vi "FRCts20_Backend_Competition_PPD_return.vi"(7 "Competition":T1, 8 "error in (no error)":errorcluster, 10 "rows affected":i32) -> (0 "error out":errorcluster, 3 "data string":string)   [LabVIEW 2014]
uses:
  FRCts20_Backend_API/FRCts20_Backend_API_Competition.ctl
  FRCts20_Backend_Engine.lvlib
  FRCts20_Backend_API/FRCts20_Backend_API.lvlib
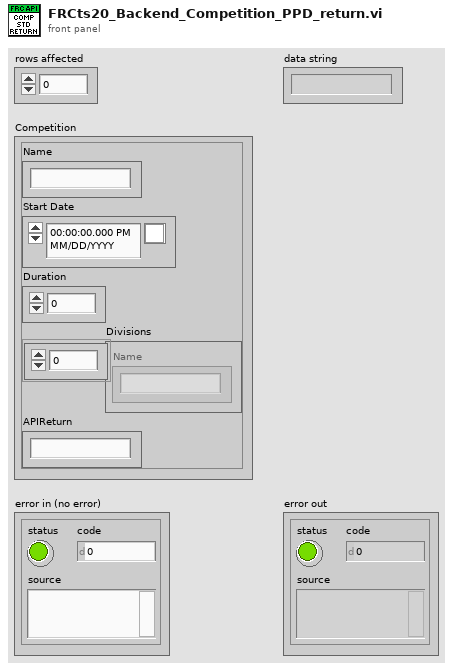
[diagram p1: front panel]
types:
  T1 = typedef "FRCts20_Backend_API.lvlib/FRCts20_Backend_API_Competition.ctl" = cluster{"Name":string, "Start Date":timestamp, "Duration":u8, "Divisions":string[], "APIReturn":string}
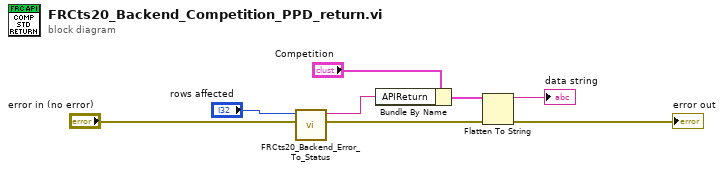
[diagram p0: block diagram]
diagram:
  n1 = call "FRCts20_Backend_Error_To_Status.vi"("error in (no error)"="error in (no error)", "rows affected"="rows affected") -> ("error out"=w4:errorcluster, "String"=w5:string)  [unwired: 8 in]
  n2 = Bundle By Name(cluster="Competition", "APIReturn"=w5) -> (w3:T1)
  n3 = Flatten To String(anything=w3, error in (no error)=w4) -> (data string=→"data string":string, error out=→"error out":errorcluster)  [unwired: 2 in, 1 out]
